vi "Field Scouting.vi"() -> ()   [LabVIEW 2016]
uses:
  <vilib>/Utility/sysdir.llb/System Directory Type.ctl
panel:
  in  "?":enum32{"Page 1", "Page 2"}(tab)
  in  "Auto?":bool
  in  "What does it do?":string
  in  "Gears 2":dbl
  in  "High Goals 2":dbl
  in  "Low Goals 2":dbl
  in  "Comments":string
  in  "?":bool
  in  "Gears":dbl
  in  "Speed":string(combo)
  in  "Low Goals":dbl
  in  "High Goals":dbl
  in  "Rating":dbl=1.0 min=1.0 max=5.0 step=0.5
  in  "Team #":string
  # "AUTONOMOUS"
  # "TELEOPERATED"
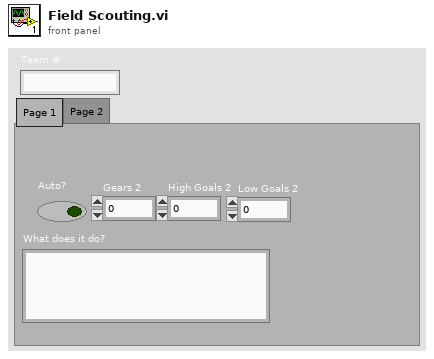
[diagram p1: front panel]
types:
  T1 = typedef "System Directory Type.ctl" = i32
  T2 = enum16{"open", "replace", "create", "open or create", "replace or create", "replace or create with confirmation"}
  T3 = enum32{"invalid app kind", "Development System", "Run Time System", "Student Edition", "Embedded LabVIEW", "Evaluation", "Custom"}
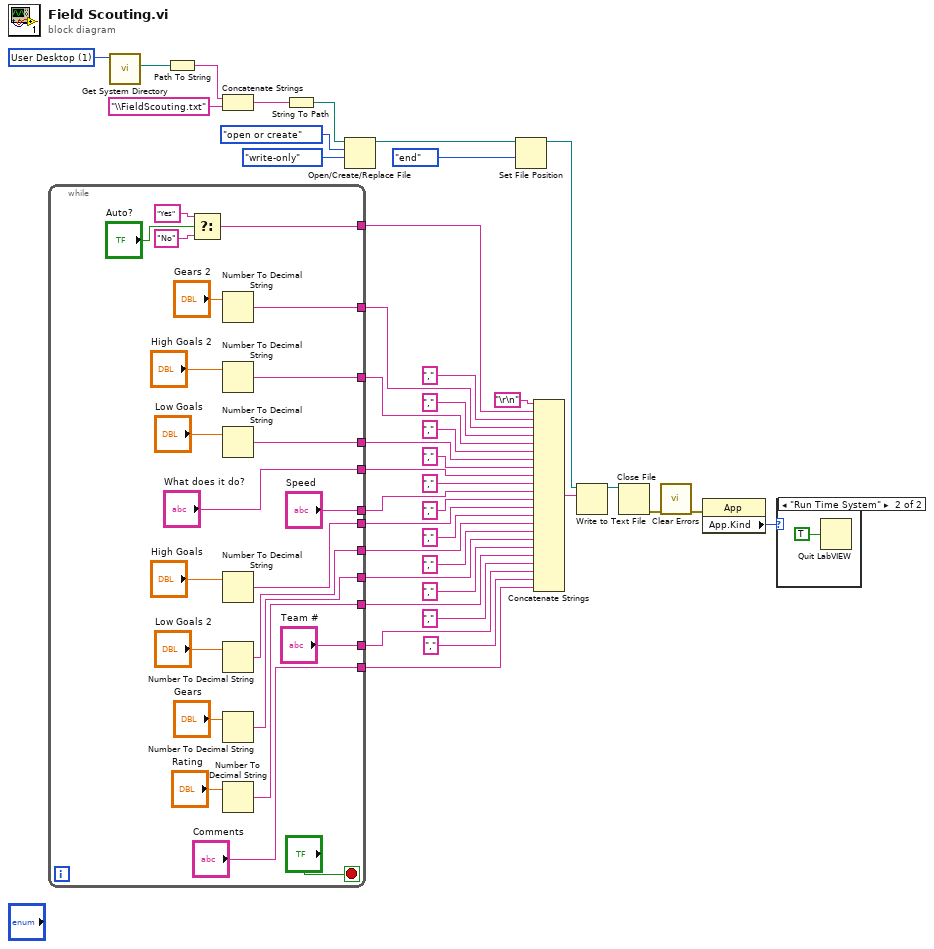
[diagram p0: block diagram]
diagram:
  w16 = T1 1 items=["User Home"=0, "User Desktop"=1, "User Documents"=2, "User Application Data"=3, "User Preferences"=4, "User Temporary"=5, "Public Documents"=6, "Public Application Data"=7, "Public Preferences"=8, "Public Cache"=13, "System Core Libraries"=9, "System Installed Libraries"=10, "Application Files"=11, "Boot Volume Root"=12] ("system directory type")
  n1 = while {
    tunnel: [w52] -> w30
    tunnel: [w51] -> w29
    tunnel: [w50] -> w28
    tunnel: [w49] -> w27
    tunnel: ["What does it do?"] -> w26
    tunnel: ["Speed"] -> w25
    tunnel: [w46] -> w24
    tunnel: [w45] -> w23
    tunnel: [w44] -> w22
    tunnel: [w43] -> w21
    tunnel: ["Team #"] -> w3
    tunnel: ["Comments"] -> w1
    stop <- "?" stop-if-true
    n2 = Select(t="Yes", s="Auto?", f="No") -> (s? t:f=w52:string)
    n3 = Number To Decimal String(number="Gears 2") -> (decimal integer string=w51:string)  [unwired: 1 in]
    n4 = Number To Decimal String(number="High Goals 2") -> (decimal integer string=w50:string)  [unwired: 1 in]
    n5 = Number To Decimal String(number="Low Goals") -> (decimal integer string=w49:string)  [unwired: 1 in]
    n6 = Number To Decimal String(number="High Goals") -> (decimal integer string=w46:string)  [unwired: 1 in]
    n7 = Number To Decimal String(number="Low Goals 2") -> (decimal integer string=w45:string)  [unwired: 1 in]
    n8 = Number To Decimal String(number="Gears") -> (decimal integer string=w44:string)  [unwired: 1 in]
    n9 = Number To Decimal String(number="Rating") -> (decimal integer string=w43:string)  [unwired: 1 in]
  }
  n10 = call <vilib>:"Get System Directory.vi"("system directory type"=w16) -> ("system directory"=w15:path)  [unwired: 10 in]
  n11 = Path To String(path=w15) -> (string=w14:string)
  n12 = Concatenate Strings(w14, "\\FieldScouting.txt" ("string")) -> (w12:string)
  n13 = String To Path(string=w12) -> (path=w11:path)
  n14 = Open/Create/Replace File(file path (use dialog)=w11, operation (0:open)=T2."open or create", access (0:read/write)=enum16{"read/write", "read-only", "write-only"}."write-only") -> (refnum out=w18:refnum<file>)  [unwired: 3 in, 2 out]
  n15 = Set File Position(refnum=w18, from (0:start)=enum16{"start", "end", "current"}."end") -> (refnum out=w6:refnum<file>)  [unwired: 2 in, 1 out]
  n16 = Concatenate Strings("\r\n", w30, ",", w29, ",", w28, ",", w27, ",", w26, ",", w25, ",", w24, ",", w23, ",", w22, ",", w21, ",", w3, ",", w1) -> (w5:string)
  n17 = Write to Text File(file (use dialog)=w6, text=w5) -> (refnum out=w10:refnum<file>)  [unwired: 2 in, 2 out]
  n18 = Close File(refnum=w10) -> (error out=w9:errorcluster)  [unwired: 1 in, 1 out]
  n19 = call <vilib>:"Clear Errors.vi"("error in (no error)"=w9) -> ("error out"=w8:errorcluster)  [unwired: 5 in, 1 out]
  n20 = property class="App"(error in=w8) -> ("App.Kind"=w7:T3)  [unwired: 1 in, 2 out]
  n21 = case shown="\"Run Time System\"" w7 {
    frame Default {
    }
    frame "Run Time System" {
      n22 = Quit LabVIEW(quit? (T)=TRUE) -> ()
    }
  }
